vi "GlobalAotfSettings.vi"() -> ()   [LabVIEW 2011]
panel:
  in  "PowerChannelAotf":i16[](array[numeric])
  in  "WavelengthAOTF":i32[](array[numeric])
  in  "LaserAOTFOnOff":bool[](array[boolean])
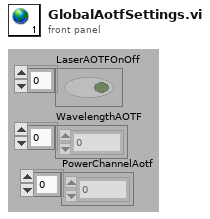
[diagram p1: front panel]
diagram:
